vi "TachoPulseGenerationTest.vi"() -> ()   [LabVIEW 2023]
uses:
  <vilib>/measure/mascope.llb/Pulse Measurements 1 chan.vi
  <vilib>/Waveform/WDTOps.llb/WDT Get Final Time Value DBL.vi
  <vilib>/Waveform/DWDTOps.llb/DWDT Analog to Digital.vi
  <vilib>/Waveform/DWDTOps.llb/DWDT Digital Size.vi
  <vilib>/measure/mamon.llb/Waveform Peak Detection for 1 Chan.vi
  <vilib>/measure/NI_MABase.lvlib
  <vilib>/measure/NI_MAPro.lvlib
panel:
  out "Pulse duration":dbl
  out "Pulse period":dbl
  out "Pulse frequency":dbl
  out "number of signals":i32
  out "number of samples":i32
  out "duty cycle":dbl format="%.2g"
  out "pulse duration":dbl format="%.2g"
  out "period":dbl format="%.2g"
  in  "width":i32=3 min=3
  in  "threshold":dbl format="%.2p"
  out "dt":dbl
  out "t0":timestamp
  out "tf":timestamp
  in  "RPM":dbl
  out "Peaks found":i32
  out "Digital Waveform Graph 2":digitalwaveform(graph)
  out "Waveform Graph":waveform(dbl)(graph)
  in  "phase":dbl format="%.2p"
  in  "amplitude":dbl=1.0 format="%0.2p"
  out "frequency":dbl=10.0 format="%0.2p"
  # "Pulse generator"
  # "Peak detection"
  # "Digital waveform info"
  # "Analog wfm pulse measurements"
  # "Analog timing measurement"
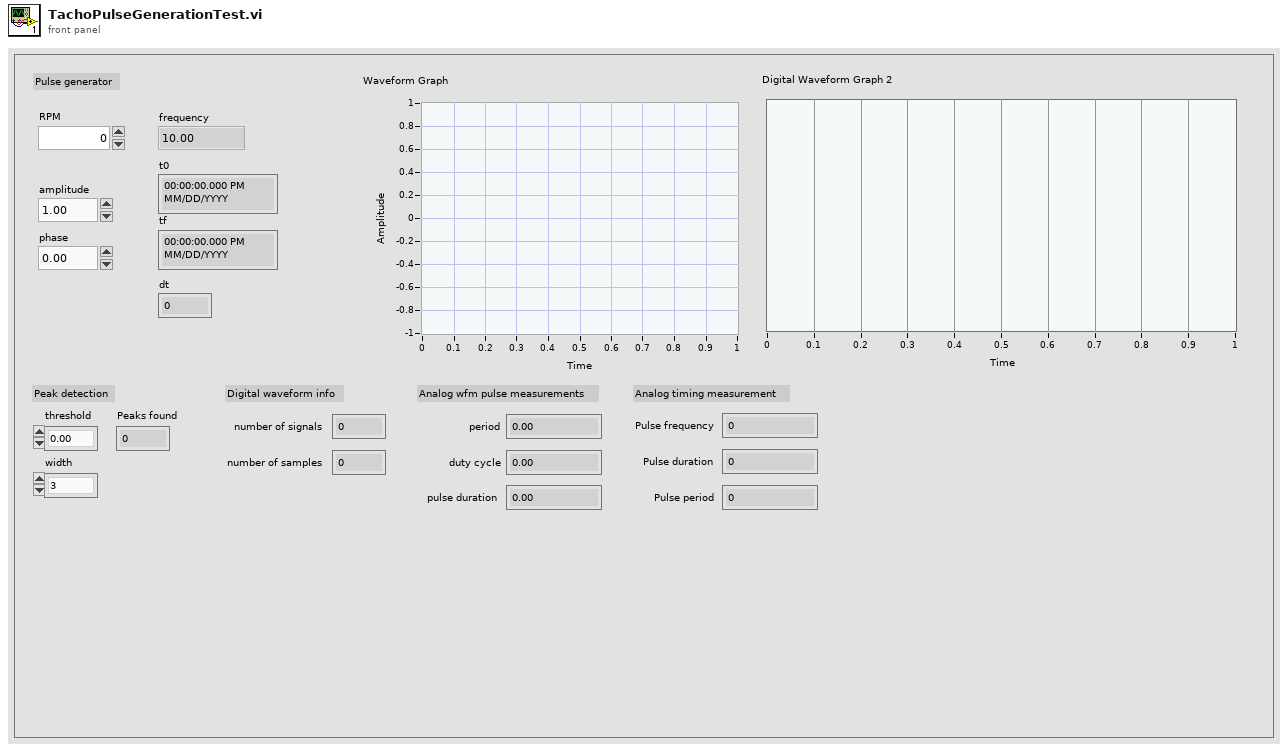
[diagram p1: front panel]
types:
  T1 = enum16{"Sine Wave", "Triangle Wave", "Square Wave", "Sawtooth Wave"}
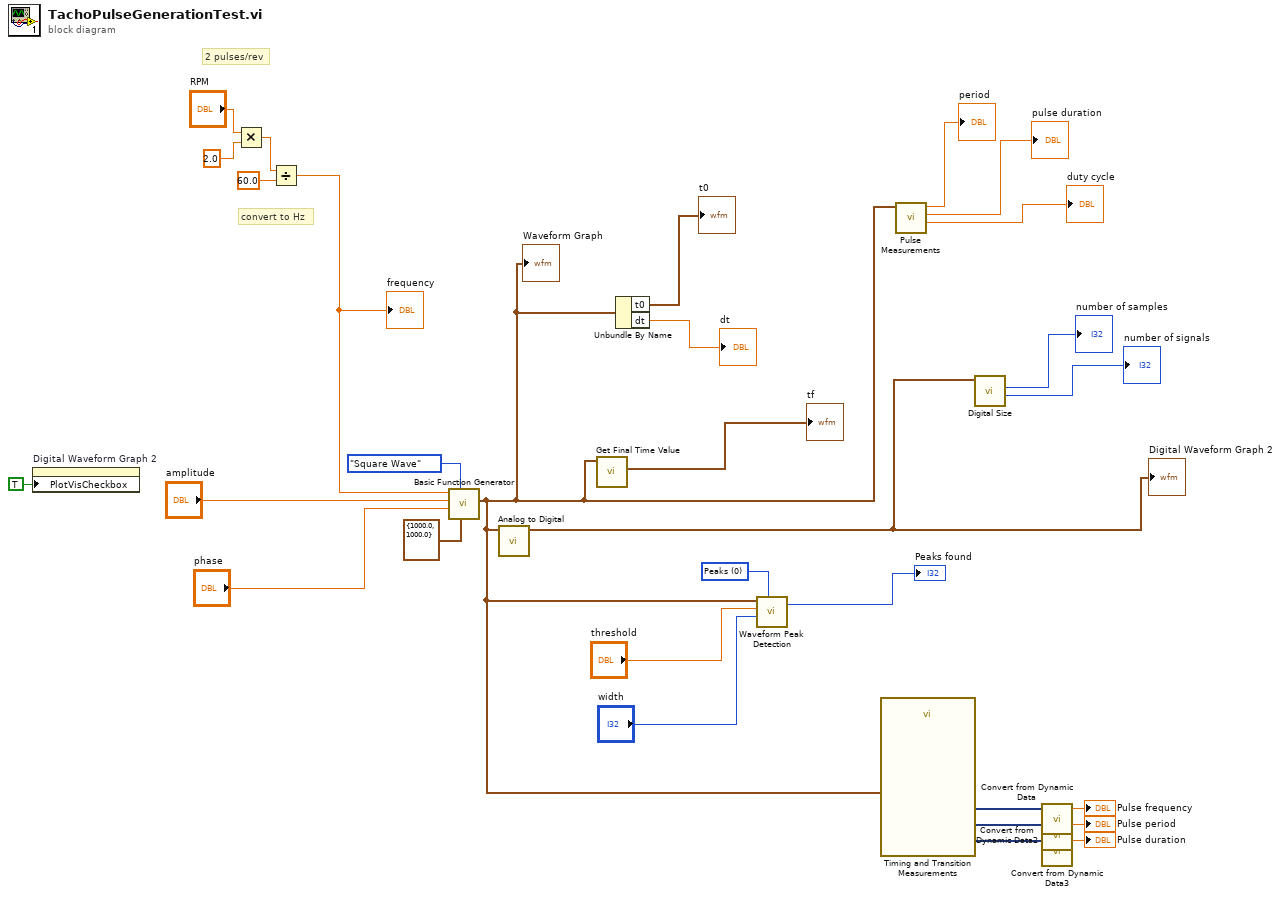
[diagram p0: block diagram]
diagram:
  w25 = u16 0 items=["Peaks", "Valleys"] ("peaks/valleys")
  # "convert to Hz"
  # "2 pulses/rev"
  n1 = property on="Digital Waveform Graph 2" class="DigitalGraph (strict)"("PlotVisCheckbox"=TRUE ("Legend:Plot Visibility Checkbox Visible")) -> ()  [unwired: 2 in, 2 out]
  n2 = Multiply(x="RPM", y=2.0) -> (x*y=w21:dbl)
  n3 = Divide(x=w21, y=60.0) -> (x/y=w19:dbl)
  "frequency" <- w19
  n4 = call <vilib>:"Basic Function Generator.vi"("sampling info"=cluster{"Fs":dbl, "#s":dbl} {"Fs"=1000.0, "#s"=1000.0}, "signal type"=T1."Square Wave", "phase"="phase", "amplitude"="amplitude", "frequency"=w19) -> ("signal out"=w7:waveform(dbl))  [unwired: 4 in, 2 out]
  "Waveform Graph" <- w7
  n5 = call-poly <vilib>:"Analog to Digital.vi"("analog waveform"=w7) -> ("digital waveform"=w8:digitalwaveform)  [unwired: 7 in, 3 out]
  "Digital Waveform Graph 2" <- w8
  n6 = call-poly <vilib>:"Get Final Time Value.vi"("waveform in"=w7) -> ("tf"=→"tf":timestamp)  [unwired: 8 in, 2 out]
  n7 = Unbundle By Name(w7) -> ("t0"=→"t0":timestamp, "dt"=→"dt":dbl)
  n8 = call-poly <vilib>:"Waveform Peak Detection.vi"("peaks/valleys"=w25, "width"="width", "threshold"="threshold", "Signal In"=w7) -> ("# found"=→"Peaks found":i32)  [unwired: 3 in, 4 out]
  n9 = call "Timing and Transition Measurements"("Signals"=w7) -> ("Frequency"=w6:dynamicdata, "Period"=w3:dynamicdata, "Duration"=w2:dynamicdata)  [unwired: 7 in, 1 out]
  n10 = call-poly <vilib>:"Pulse Measurements.vi"("signal in"=w7) -> ("duty cycle"=→"duty cycle":dbl, "pulse duration"=→"pulse duration":dbl, "period"=→"period":dbl)  [unwired: 6 in, 2 out]
  n11 = call-poly <vilib>:"Digital Size.vi"("digital waveform in"=w8) -> ("number of signals"=→"number of signals":i32, "number of samples"=→"number of samples":i32)  [unwired: 7 in, 2 out]
  n12 = call "Convert from Dynamic Data"("Dynamic Data Type"=w6) -> ("Scalar"=→"Pulse frequency":dbl)  [unwired: 3 in]
  n13 = call "Convert from Dynamic Data2"("Dynamic Data Type"=w3) -> ("Scalar"=→"Pulse period":dbl)  [unwired: 3 in]
  n14 = call "Convert from Dynamic Data3"("Dynamic Data Type"=w2) -> ("Scalar"=→"Pulse duration":dbl)  [unwired: 3 in]
